vi "WLAN Tx Test Set WLAN INSTR TX.vi"(8 "error in (no error)":errorcluster, 10 "niDTS WLAN.lvlib:niDTS WLAN INSTR TX":refnum<class "niDTS WLAN INSTR TX.lvclass">, 11 "niDTS WLAN Tx Test in":refnum<class "niDTS WLAN Tx Test.lvclass">) -> (0 "error out":errorcluster, 3 "niDTS WLAN Tx Test out":refnum<class "niDTS WLAN Tx Test.lvclass">)   [LabVIEW 2015, in "niDTS WLAN.lvlib" / "niDTS WLAN Tx Test.lvclass"]
uses:
  niDTS WLAN Tx Test.lvclass
  Instrument/INSTR TX/niDTS WLAN INSTR TX.lvclass
  niDTS WLAN Tx Test.lvclass/niDTS WLAN Tx Test.ctl
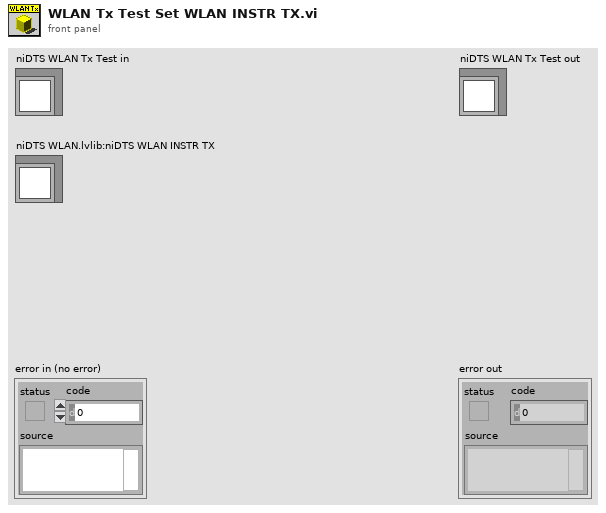
[diagram p1: front panel]
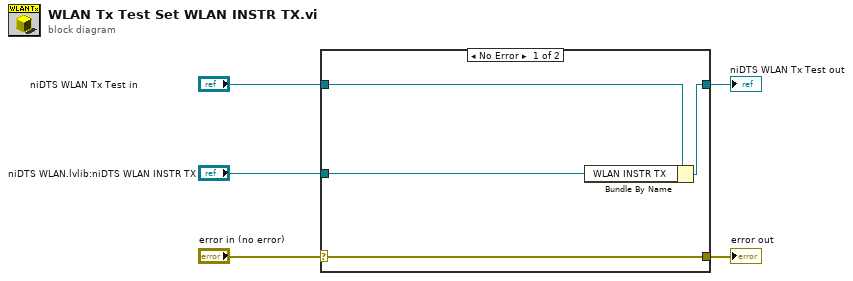
[diagram p0: block diagram]
diagram:
  n1 = case shown="No Error" "error in (no error)" {
    selector: "error in (no error)" -> [w9 w10]
    tunnel: [w9 w10] -> w4
    tunnel: [w7 w11] -> w2
    tunnel: "niDTS WLAN Tx Test in" -> [w8 w11]
    tunnel: "niDTS WLAN.lvlib:niDTS WLAN INSTR TX" -> [w6 _]
    frame No Error {
      n2 = Bundle By Name(cluster=w8, "WLAN INSTR TX"=w6) -> (w7:refnum<class "niDTS WLAN Tx Test.lvclass">)
    }
    frame Error {
    }
  }
  "error out" <- w4
  "niDTS WLAN Tx Test out" <- w2
